vi "Log Framework Event.vi"(7 "Event Level (Debug)":T1, 8 "error in (no error)":errorcluster, 9 "Data To Log":string, 11 "IMediator In":refnum<class "IMediator.lvclass">) -> (0 "error out":errorcluster)   [LabVIEW 2020, in "IMediator.lvlib" / "IMediator.lvclass"]
uses:
  <vilib>/gpm_packages/@cs/mva-core/Source/IMediator/IMediator/IMediator.lvclass
  <vilib>/gpm_packages/@cs/event-logger/Source/Composed Log/Types/Log Level.ctl
  <vilib>/gpm_packages/@cs/mva-core/Source/IMediator/IMediator/IMediator.lvclass/IMediator.ctl
  <vilib>/gpm_packages/@cs/event-logger/Source/Composed Log/LoggerReference/LoggerReference.lvclass/LoggerReference.ctl
  <vilib>/gpm_packages/@cs/event-logger/Source/Composed Log/LoggerReference/Log.vi
  <vilib>/gpm_packages/@cs/event-logger/Source/Composed Log/LoggerReference/Get Valid Event Time.vi
  <vilib>/gpm_packages/@cs/event-logger/Source/Composed Log/LoggerReference/Remove Stale Logs.vi
  <vilib>/gpm_packages/@cs/event-logger/Source/Composed Log/LoggerReference/LoggerReference.lvclass
  <vilib>/gpm_packages/@cs/event-logger/Source/Composed Log/Composed Log.lvlib
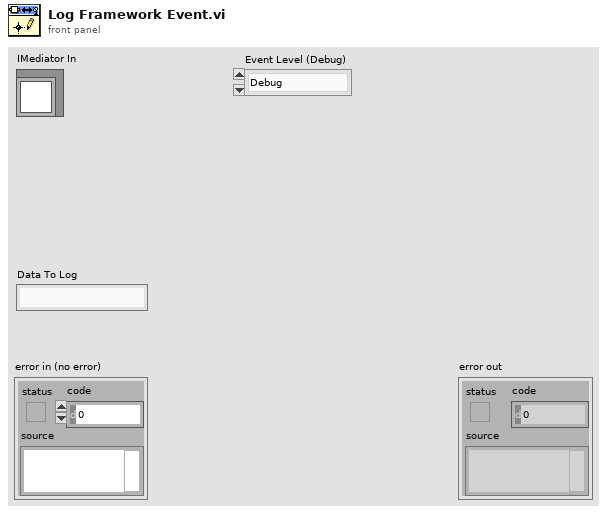
[diagram p1: front panel]
types:
  T1 = typedef "Composed Log.lvlib/Log Level.ctl" = enum16{"Debug", "Info", "Warning", "Error", "Critical"}
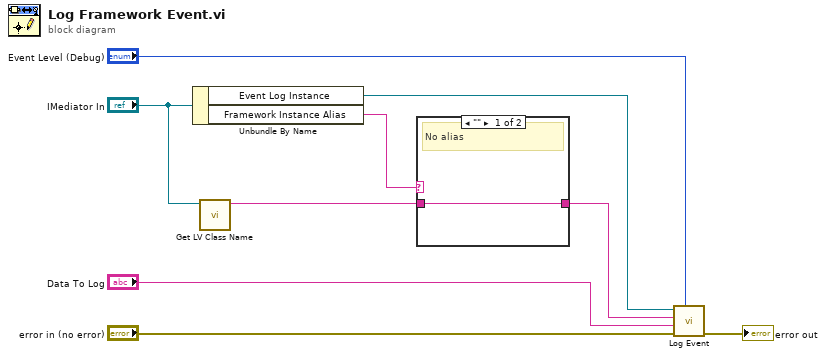
[diagram p0: block diagram]
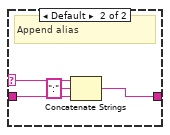
[diagram p2: hidden frame]
diagram:
  n1 = Unbundle By Name("IMediator In") -> ("Event Log Instance"=w7:refnum<class "LoggerReference.lvclass">, "Framework Instance Alias"=w1:string)
  n2 = call <vilib>:"Get LV Class Name.vi"("object"="IMediator In") -> ("class name"=w3:string)  [unwired: 9 in, 1 out]
  n3 = case shown="\"\"" w1 {
    selector: w1 -> [_ w14]
    tunnel: [w10 w13] -> w2
    tunnel: w3 -> [w10 w12]
    frame "" {
      # "No alias"
    }
    frame Default {
      # "Append alias"
      n4 = Concatenate Strings(w14, ":" ("string"), w12) -> (w13:string)
    }
  }
  n5 = call <vilib>:"Log Event.vi"("Event Level"="Event Level (Debug)", "error in (no error)"="error in (no error)", "Data To Log"="Data To Log", "SourceID"=w2, "Log Instance"=w7) -> ("error out"=→"error out":errorcluster)  [unwired: 5 in, 1 out]
